vi "NotifyIcon - Get All MenuItems.vi"(8 "error in (no error)":errorcluster, 9 "MenuItem references in":refnum<k24>[](array[refnum]), 11 "MenuItem Collection reference":refnum<k24>) -> (0 "error out":errorcluster, 1 "MenuItem references out":refnum<k24>[](array[refnum]))   [LabVIEW 2015]
doc: "Recursive"
uses:
  System.Windows.Forms
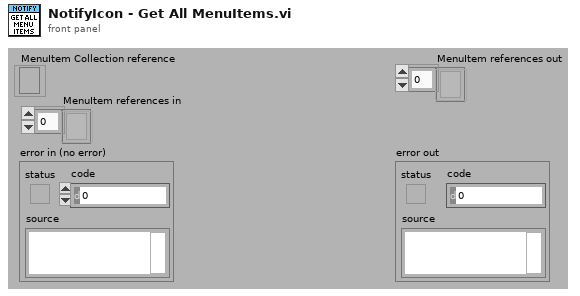
[diagram p1: front panel]
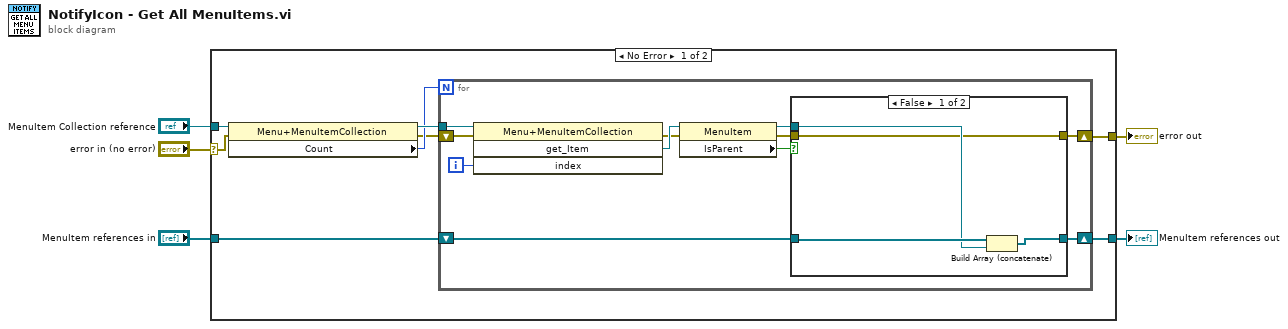
[diagram p0: block diagram]
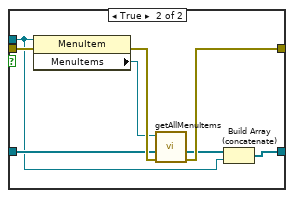
[diagram p2: hidden frame]
diagram:
  n1 = case shown="No Error" "error in (no error)" {
    selector: "error in (no error)" -> [w6 w38]
    tunnel: "MenuItem references in" -> [w11 w37]
    tunnel: "MenuItem Collection reference" -> [w10 _]
    tunnel: [w9 w37] -> w3
    tunnel: [w7 w38] -> w2
    frame No Error {
      n2 = property class="Menu+MenuItemCollection"(reference=w10, error in=w6) -> (reference out=w13:refnum<k24>, error out=w8:errorcluster, "Count"=w12:i32)
      n3 = for {
        N: w12 -> [_]
        tunnel: w13 -> [w24]
        shift-right: [w20] -> w9
        shift-left: w11 -> [w19]
        shift-right: [w14] -> w7
        shift-left: w8 -> [w17]
        i -> [w21]
        n4 = invoke class="Menu+MenuItemCollection" method="get_Item"(reference=w24, error in=w17, "index"=w21) -> (error out=w16:errorcluster, "get_Item"=w22:refnum<k24>)  [unwired: 1 in, 2 out]
        n5 = property class="MenuItem"(reference=w22, error in=w16) -> (reference out=w18:refnum<k24>, error out=w15:errorcluster, "IsParent"=w23:bool)
        n6 = case shown="False" w23 {
          tunnel: [w28 w30] -> w20
          tunnel: w19 -> [w27 w35]
          tunnel: w18 -> [w26 w31]
          tunnel: w15 -> [w25 w34]
          tunnel: [w25 w33] -> w14
          frame False {
            n7 = Build Array (concatenate)(w27, w26) -> (w28:refnum<k24>[])
          }
          frame True {
            n8 = property class="MenuItem"(reference=w31, error in=w34) -> (error out=w36:errorcluster, "MenuItems"=w29:refnum<k24>)  [unwired: 1 out]
            n9 = call "getAllMenuItems.vi"("error in (no error)"=w36, "MenuItem references in"=w35, "MenuItem Collection reference"=w29) -> ("error out"=w33:errorcluster, "MenuItem references out"=w32:refnum<k24>[])  [unwired: 7 in]
            n10 = Build Array (concatenate)(w32, w31) -> (w30:refnum<k24>[])
          }
        }
      }
    }
    frame Error {
    }
  }
  "MenuItem references out" <- w3
  "error out" <- w2
